vi "Write_value_to_OPC.vi"(9 "Data in":variant, 10 "Address to write":string, 11 "OPC UA client refnum in":T1) -> (3 "OPC UA client refnum out":T1)   [LabVIEW 2021]
uses:
  <vilib>/OPCUA/controls/OPC UA Client Refnum.ctl
  <vilib>/OPCUA/controls/Write Status.ctl
  <vilib>/OPCUA/client/Multiple Write Variant.vi
  <vilib>/OPCUA/NI OPC UA Client.lvlib
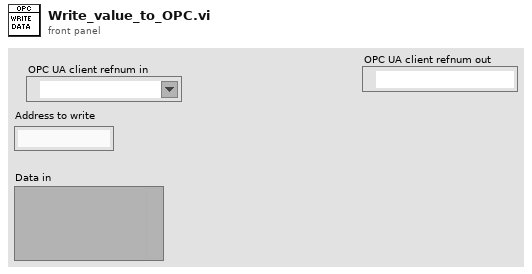
[diagram p1: front panel]
types:
  T1 = typedef "OPC UA Client Refnum.ctl" = refnum<k21>
  T2 = typedef "Write Status.ctl" = u32
  T3 = cluster{"Address to write":string, "Data in":variant, "seconds since 1Jan1904":timestamp, "node status":T2}
  T4 = cluster{"Address to write":string, "Data in":variant, "seconds since 1Jan1904":timestamp, "node status":T2}[]
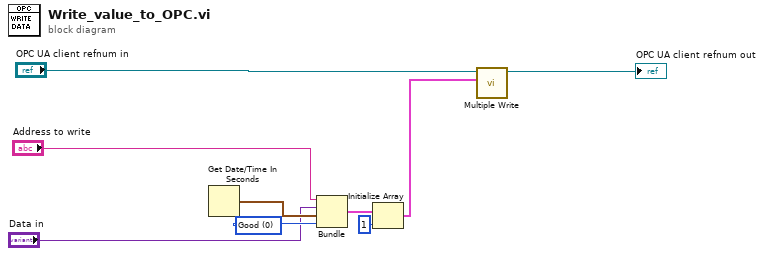
[diagram p0: block diagram]
diagram:
  w7 = T2 0 items=["Good"=0, "Uncertain"=1073741824, "Uncertain_InitialValue"=1083310080, "Uncertain_LastUsableValue"=1083179008, "Uncertain_SensorNotAccurate"=1083375616, "Uncertain_EngineeringUnitsExceeded"=1083441152, "Bad"=2147483648, "Bad_NoCommunication"=2150694912, "Bad_NotReadable"=2151284736, "Bad_NotWritable"=2151350272, "Bad_OutOfRange"=2151415808, "Bad_WaitingForInitialData"=2150760448] ("node status")
  n1 = Get Date/Time In Seconds() -> (seconds since 1Jan1904=w4:timestamp)
  n2 = Bundle("Address to write"="Address to write", "Data in"="Data in", "seconds since 1Jan1904"=w4, "node status"=w7) -> (w6:T3)  [unwired: 1 in]
  n3 = Initialize Array(w6, 1 ("dimension size")) -> (w2:T4)
  n4 = call-poly <vilib>:"Multiple Write.vi"("requests"=w2, "OPC UA client refnum in"="OPC UA client refnum in") -> ("OPC UA client refnum out"=→"OPC UA client refnum out":T1)  [unwired: 6 in, 3 out]
